vi "Get Last Row.vi"(8 "error in (no error)":errorcluster, 10 "Sheet Reference":refnum<k24>) -> (0 "error out":errorcluster, 2 "Sheet Reference out":refnum<k24>, 5 "Last Row":i32)   [LabVIEW 2013]
doc: "Returns the last row. This number is zero-based."
uses:
  C:/PhaeronGit/LVNPOI/Resources/NPOI 2.1.1 dotnet2/NPOI.dll
  Resources/NPOI 2.1.1 dotnet2/NPOI.dll
panel:
  # "This is zero-based."
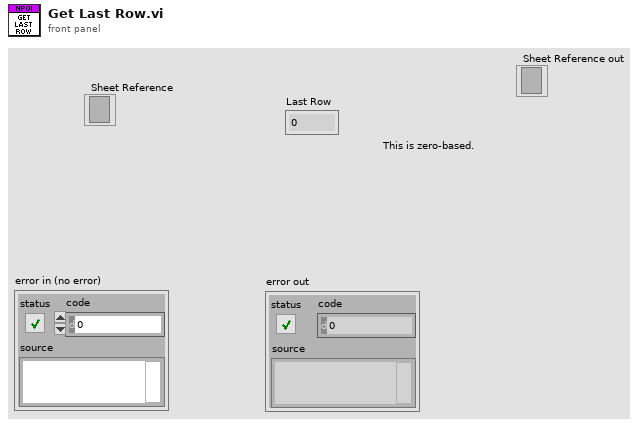
[diagram p1: front panel]
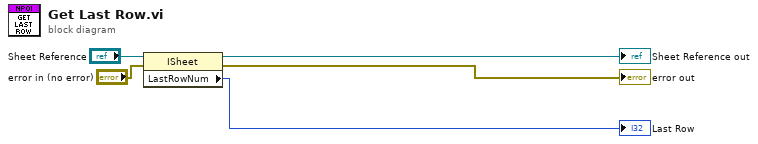
[diagram p0: block diagram]
diagram:
  n1 = property class="ISheet"(reference="Sheet Reference", error in="error in (no error)") -> (reference out=→"Sheet Reference out":refnum<k24>, error out=→"error out":errorcluster, "LastRowNum"=→"Last Row":i32)
